vi "Find All Uses.Highlight Node.vi"(11 "Node in":refnum<vi>) -> ()   [LabVIEW 2020]
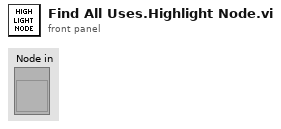
[diagram p1: front panel]
types:
  T1 = enum32{"Invalid", "Standard", "Closed", "Hidden", "Minimized", "Maximized"}
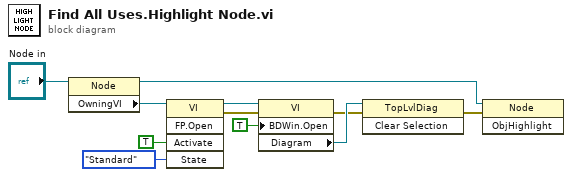
[diagram p0: block diagram]
diagram:
  n1 = property class="Node"(reference="Node in") -> (reference out=w7:refnum<vi>, "OwningVI"=w1:refnum<vi>)  [unwired: 1 in, 1 out]
  n2 = invoke class="VI" method="FP.Open"(reference=w1, "Activate"=TRUE ("Activate?"), "State"=T1."Standard") -> (reference out=w4:refnum<vi>, error out=w5:errorcluster)  [unwired: 2 in, 3 out]
  n3 = property class="VI"(reference=w4, error in=w5, "BDWin.Open"=TRUE ("Block Diagram Window:Open")) -> (error out=w9:errorcluster, "Diagram"=w11:refnum<vi>)  [unwired: 1 out]
  n4 = invoke class="TopLvlDiag" method="Clear Selection"(reference=w11, error in=w9) -> (error out=w10:errorcluster)  [unwired: 1 in, 2 out]
  n5 = invoke class="Node" method="ObjHighlight"(reference=w7, error in=w10) -> ()  [unwired: 1 in, 3 out]
